vi "CRYPIC GET FRAME.vi"(10 "nID":i32) -> (0 "tFrame_Out":T2, 1 "sData_Out":string, 2 "nID_Out":i32)   [LabVIEW 2013]
uses:
  <vilib>/Utility/miscctls.llb/LVRectTypeDef.ctl
  CRYMain Sub Window Global.vi
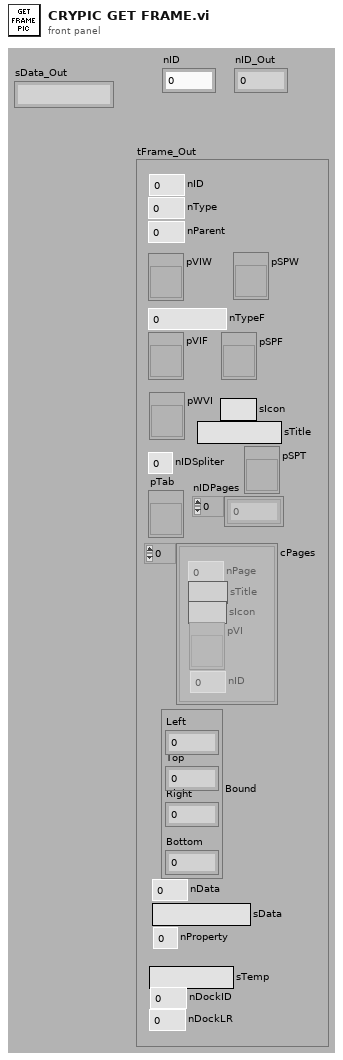
[diagram p1: front panel]
types:
  T1 = typedef "LVRectTypeDef.ctl" = cluster{"Left":i16, "Top":i16, "Right":i16, "Bottom":i16}
  T2 = cluster{"nType":i32, "nParent":i32, "pVIW":refnum<vi>, "pSPW":refnum<vi>, "nTypeF":i32, "pVIF":refnum<vi>, "pSPF":refnum<vi>, "nIDSpliter":i32, "nProperty":i32, "Bound":T1, "nID":i32, "nData":i32, "sData":string, "pWVI":refnum<vi>, "sTitle":string, "cPages":cluster{"nPage":i32, "sTitle":string, "sIcon":string, "pVI":refnum<vi>, "nID":i32}[], "pTab":refnum<vi>, "nIDPages":i32[], "pSPT":refnum<vi>, "sTemp":string, "nDockID":i32, "nDockLR":i32, "sIcon":string}
  T3 = cluster{"nID":i32[], "Frame":cluster{"nType":i32, "nParent":i32, "pVIW":refnum<vi>, "pSPW":refnum<vi>, "nTypeF":i32, "pVIF":refnum<vi>, "pSPF":refnum<vi>, "nIDSpliter":i32, "nProperty":i32, "Bound":T1, "nID":i32, "nData":i32, "sData":string, "pWVI":refnum<vi>, "sTitle":string, "cPages":cluster{"nPage":i32, "sTitle":string, "sIcon":string, "pVI":refnum<vi>, "nID":i32}[], "pTab":refnum<vi>, "nIDPages":i32[], "pSPT":refnum<vi>, "sTemp":string, "nDockID":i32, "nDockLR":i32, "sIcon":string}[]}
  T4 = cluster{"nType":i32, "nParent":i32, "pVIW":refnum<vi>, "pSPW":refnum<vi>, "nTypeF":i32, "pVIF":refnum<vi>, "pSPF":refnum<vi>, "nIDSpliter":i32, "nProperty":i32, "Bound":T1, "nID":i32, "nData":i32, "sData":string, "pWVI":refnum<vi>, "sTitle":string, "cPages":cluster{"nPage":i32, "sTitle":string, "sIcon":string, "pVI":refnum<vi>, "nID":i32}[], "pTab":refnum<vi>, "nIDPages":i32[], "pSPT":refnum<vi>, "sTemp":string, "nDockID":i32, "nDockLR":i32, "sIcon":string}[]
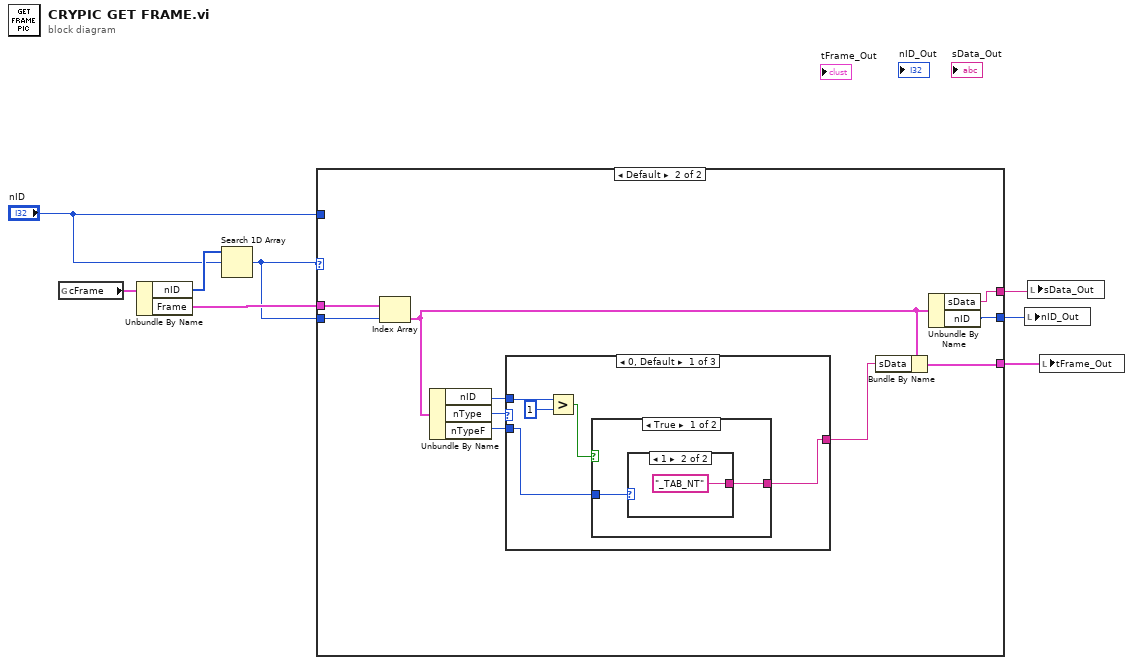
[diagram p0: block diagram]
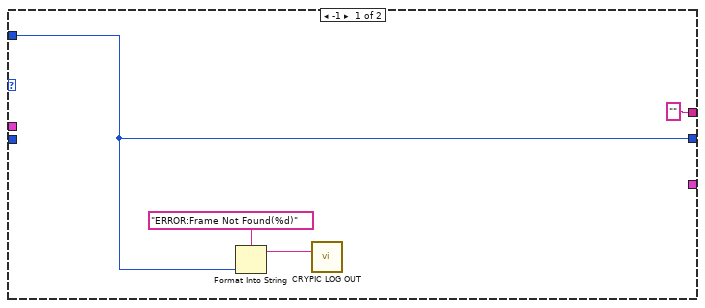
[diagram p2: hidden frame]
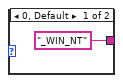
[diagram p3: hidden frame]
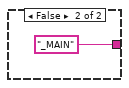
[diagram p4: hidden frame]
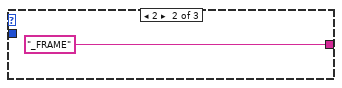
[diagram p5: hidden frame]
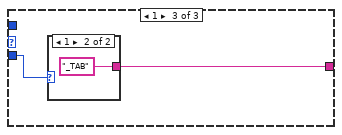
[diagram p6: hidden frame]
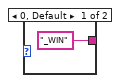
[diagram p7: hidden frame]
diagram:
  n1 = global read "CRYMain Sub Window Global.vi" "cFrame"() -> (w6:T3)
  n2 = Unbundle By Name(w6) -> ("nID"=w8:i32[], "Frame"=w7:T4)
  n3 = Search 1D Array(1D array=w8, element="nID") -> (index of element=w5:i32)  [unwired: 1 out]
  n4 = case shown="Default" w5 {
    tunnel: w7 -> [_ w22]
    tunnel: w5 -> [_ w18]
    tunnel: "nID" -> [w10 _]
    tunnel: [_ w14] -> w3
    tunnel: [w10 w17] -> w2
    tunnel: ["" ("sData_Out") w13] -> w1
    frame -1 {
      n5 = Format Into String(format string="ERROR:Frame Not Found(%d)", w10) -> (resulting string=w11:string)  [unwired: 2 in, 1 out]
      n6 = call "CRYPIC LOG OUT.vi"("sData"=w11) -> ()  [unwired: 11 in]
    }
    frame Default {
      n7 = Index Array(array=w22, index=w18) -> (element=w16:T2)
      n8 = Unbundle By Name(w16) -> ("nID"=w19:i32, "nType"=w21:i32, "nTypeF"=w20:i32)
      n9 = case shown="0, Default" w21 {
        tunnel: w20 -> [w25 _ w35]
        tunnel: [w26 "_FRAME" ("sData_Out") w34] -> w15
        tunnel: w19 -> [w24 _ _]
        frame 0, Default {
          n10 = Greater?(x=w24, y=1) -> (0:w27:bool)
          n11 = case shown="True" w27 {
            tunnel: [w28 "_MAIN" ("sData_Out")] -> w26
            tunnel: w25 -> [w29 _]
            frame True {
              n12 = case shown="1" w29 {
                tunnel: ["_WIN_NT" ("sData_Out") "_TAB_NT" ("sData_Out")] -> w28
                frame 0, Default {
                }
                frame 1 {
                }
              }
            }
            frame False {
            }
          }
        }
        frame 2 {
        }
        frame 1 {
          n13 = case shown="1" w35 {
            tunnel: ["_WIN" ("sData_Out") "_TAB" ("sData_Out")] -> w34
            frame 0, Default {
            }
            frame 1 {
            }
          }
        }
      }
      n14 = Bundle By Name(cluster=w16, "sData"=w15) -> (w14:T2)
      n15 = Unbundle By Name(w16) -> ("sData"=w13:string, "nID"=w17:i32)
    }
  }
  n16 = local write "nID_Out"(w2) -> ()
  n17 = local write "sData_Out"(w1) -> ()
  n18 = local write "tFrame_Out"(w3) -> ()
